vi "insert anything tests.vi"() -> ()   [LabVIEW 2016]
uses:
  API/JSON Document Class/json to string/json To Minimized String - string path.vi
  API/JSON Document Class/JSON Document.lvclass
panel:
  out "replaced?":bool
  in  "Cluster":T1
  out "json string":string
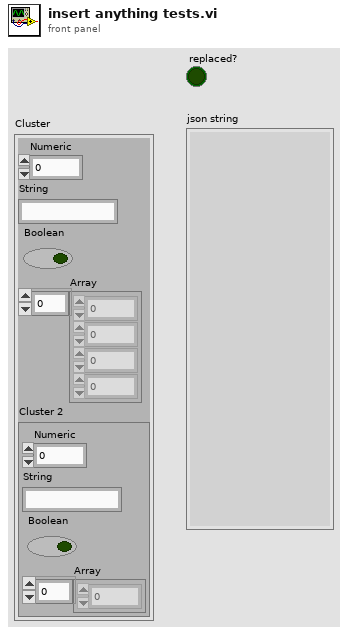
[diagram p1: front panel]
types:
  T1 = cluster{"Numeric":dbl, "String":string, "Boolean":bool, "Array":dbl[], "Cluster 2":cluster{"Numeric":dbl, "String":string, "Boolean":bool, "Array":dbl[]}}
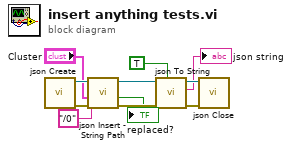
[diagram p0: block diagram]
diagram:
  n1 = call "json Create.vi"() -> ("error out"=w5:errorcluster, "JSON Document out"=w4:refnum<class "JSON Document.lvclass">)  [unwired: 10 in]
  n2 = call "json Insert - String Path.vi"("error in (no error)"=w5, "anything"="Cluster", "path"="/0", "JSON Document in"=w4) -> ("error out"=w10:errorcluster, "replaced?"=→"replaced?":bool, "JSON Document out"=w11:refnum<class "JSON Document.lvclass">)  [unwired: 5 in]
  n3 = call-poly "json To String.vi"("pretty print?"=TRUE, "error in (no error)"=w10, "JSON Document in"=w11) -> ("error out"=w7:errorcluster, "json string"=→"json string":string, "JSON Document out"=w8:refnum<class "JSON Document.lvclass">)  [unwired: 6 in]
  n4 = call "json Close.vi"("error in (no error)"=w7, "JSON Document in"=w8) -> ()  [unwired: 9 in, 1 out]
